vi "Read PatternSRC.vi"(8 "error in (no error)":errorcluster, 11 "BML_Root in":refnum<class "BML_Root.lvclass">) -> (0 "error out":errorcluster, 2 "PatternSRC":string, 3 "BML_Root out":refnum<class "BML_Root.lvclass">)   [LabVIEW 2016, in "BML_Root.lvclass"]
uses:
  BML_Root.lvclass
  BML_Root.lvclass/BML_Root.ctl
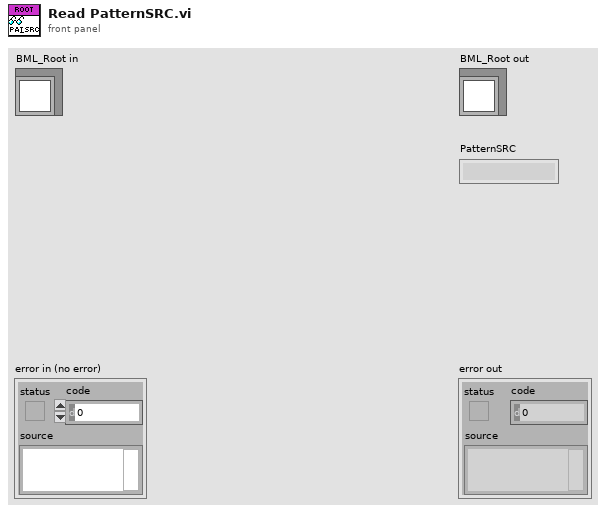
[diagram p1: front panel]
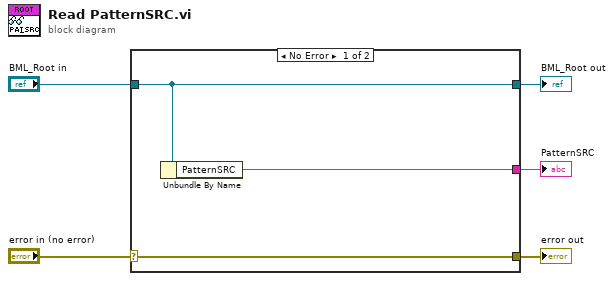
[diagram p0: block diagram]
diagram:
  n1 = case shown="No Error" "error in (no error)" {
    selector: "error in (no error)" -> [w8 w9]
    tunnel: [w8 w9] -> w4
    tunnel: [w7 w10] -> w2
    tunnel: "BML_Root in" -> [w7 w10]
    tunnel: [w6 _] -> w1
    frame No Error {
      n2 = Unbundle By Name(w7) -> ("PatternSRC"=w6:string)
    }
    frame Error {
    }
  }
  "error out" <- w4
  "BML_Root out" <- w2
  "PatternSRC" <- w1
